vi "Lvi Read U16Data2D.vi"(0 "DataBufSize":u32, 1 "timeout":dbl, 5 "TaskRef":i32, 7 "PointsPerChan":u32, 9 "NumChansToRead":u32, 11 "error in (no error)":errorcluster, 12 "OnlyReadAvailable":bool) -> (3 "DataBuf":u16[](array[numeric]), 4 "DataBufSize out":u32, 6 "TaskRef out":i32, 8 "PointsPerChan out":u32, 10 "NumChansToRead out":u32, 14 "function return":i32, 15 "error out":errorcluster)   [LabVIEW 2016, in "DtLvLink.lvlib"]
doc: "Calls directly into the entry points of the DLL of the Data Acq SDK to return a two-dimensional array of unsigned, 16-bit integers representing the data points from the specified task. \n\n\n\n\n\n\nLvErrorCode LviReadI16Data2D(unsigned int *DataBufSize, short *DataBuf, LvTaskRef * TaskRef,\n unsigned int *PointsPerChan, unsigned int *NumChansToRead, \n double timeout, bool OnlyReadAvailable);"
uses:
  <userlib>/LV-Link3/DtLvLink.lvlib
  <userlib>/LV-Link3/DtLvLink_32.dll
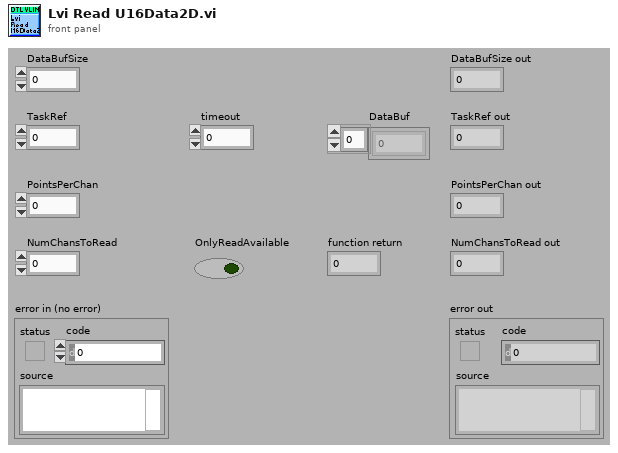
[diagram p1: front panel]
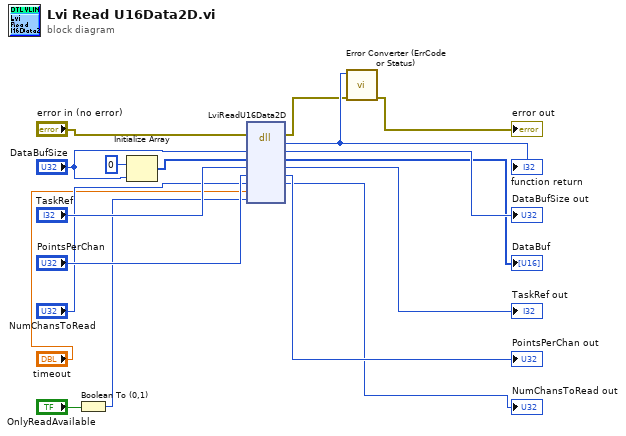
[diagram p0: block diagram]
diagram:
  n1 = Boolean To (0,1)(Boolean="OnlyReadAvailable") -> (0, 1=w4:i16)
  n2 = Initialize Array(u16 0 ("element"), "DataBufSize") -> (w15:u16[])
  n3 = dll-call lib="C:/Program Files (x86)/National Instruments/LabVIEW 2016/user.lib/LV-Link3/DtLvLink_32.*" fn="LviReadU16Data2D"(error in="error in (no error)", "DataBufSize"="DataBufSize", "DataBuf"=w15, "TaskRef"="TaskRef", "PointsPerChan"="PointsPerChan", "NumChansToRead"="NumChansToRead", "timeout"="timeout", "OnlyReadAvailable"=w4) -> (error out=w2:errorcluster, "return type"=w18:i32, "DataBufSize"=→"DataBufSize out":u32, "DataBuf"=→"DataBuf":u16[], "TaskRef"=→"TaskRef out":i32, "PointsPerChan"=→"PointsPerChan out":u32, "NumChansToRead"=→"NumChansToRead out":u32)  [unwired: 4 in, 1 out]
  "function return" <- w18
  n4 = call <userlib>:"Error Converter (ErrCode or Status).vi"("error in (no error)"=w2, "error code"=w18) -> ("error out"=→"error out":errorcluster)  [unwired: 9 in]
